vi "Update Map.vi"(8 "Direction":T1, 9 "Action":T2, 10 "Old Position":T4, 11 "Map in":T3[][](array[typedef])) -> (3 "Map out":T3[][](array[typedef]))   [LabVIEW 2020, in "Common.lvlib"]
uses:
  Common.lvlib
  Position.ctl
  Location Data.ctl
  Type Defs/Action Enum.ctl
  Type Defs/Direction Enum.ctl
  SubVIs/Read-Only Globals.vi
  Square/Board Size.vi
  SubVIs/Globals (private).vi
  Square/Square.lvclass
  Type Defs/SB Type Defs.lvlib
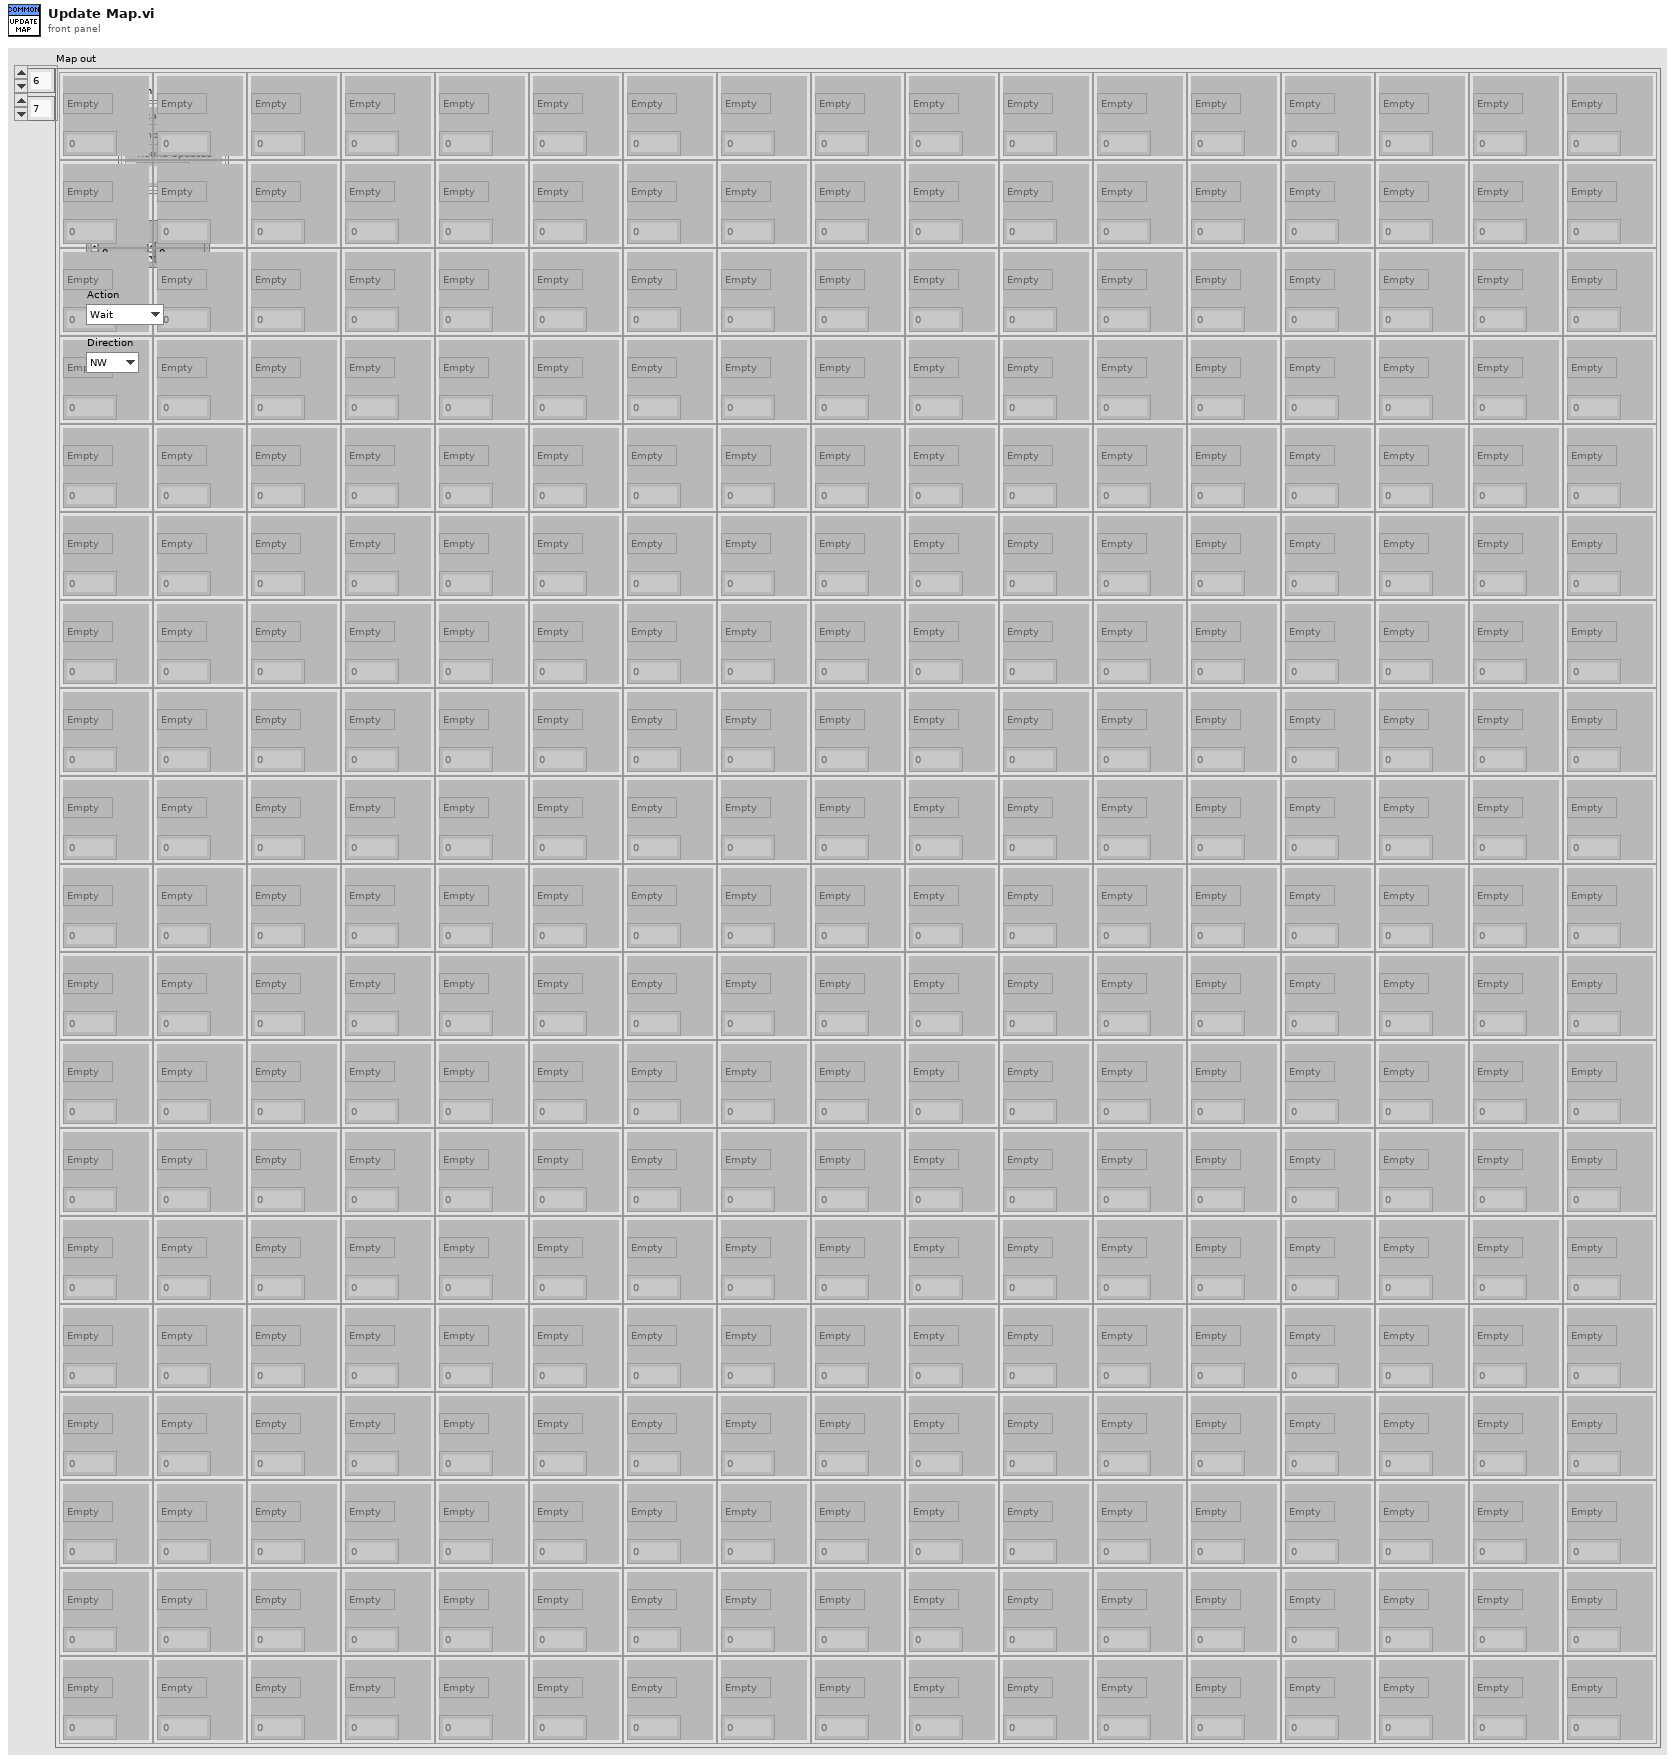
[diagram p1: front panel]
types:
  T1 = typedef "SB Type Defs.lvlib/Direction Enum.ctl" = enum16{"NW", "N", "NE", "E", "SE", "S", "SW", "W"}
  T2 = typedef "SB Type Defs.lvlib/Action Enum.ctl" = enum16{"Wait", "Move", "Attack", "Replicate"}
  T3 = typedef "Common.lvlib/Location Data.ctl" = cluster{"Location State":enum16{"Empty", "Enemy", "Attacked", "Occupied"}, "Round Updated":i32}
  T4 = typedef "Common.lvlib/Position.ctl" = cluster{"Column":i32, "Row":i32}
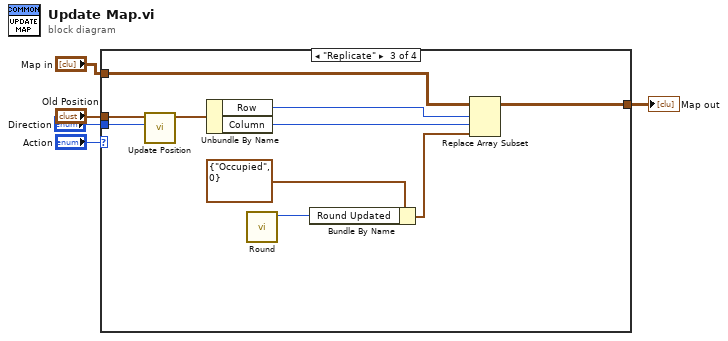
[diagram p0: block diagram]
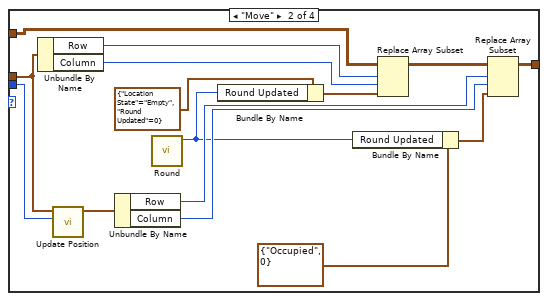
[diagram p3: hidden frame]
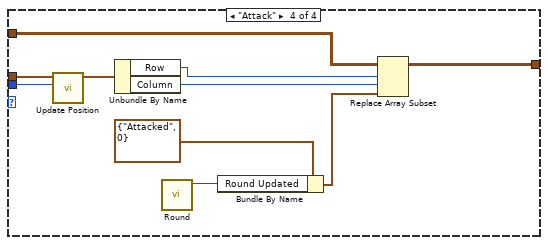
[diagram p4: hidden frame]
diagram:
  n1 = case shown="\"Replicate\"" "Action" {
    tunnel: "Old Position" -> [_ w11 w26 w36]
    tunnel: "Map in" -> [w6 w16 w29 w39]
    tunnel: [w6 w15 w28 w38] -> w3
    tunnel: "Direction" -> [_ w10 w24 w34]
    frame "Wait" {
    }
    frame "Move" {
      n2 = Unbundle By Name(w11) -> ("Row"=w21:i32, "Column"=w20:i32)
      n3 = call "Update Position.vi"("Direction"=w10, "Position in"=w11) -> ("Position out"=w12:T4)  [unwired: 9 in]
      n4 = Unbundle By Name(w12) -> ("Row"=w19:i32, "Column"=w18:i32)
      n5 = call "Round.vi"() -> ("Round"=w7:i32)  [unwired: 11 in]
      n6 = Bundle By Name(cluster=T3 {"Location State"=enum."Empty", "Round Updated"=0} ("new element/subarray"), "Round Updated"=w7) -> (w9:T3)
      n7 = Bundle By Name(cluster=T3 {"Location State"=enum."Occupied", "Round Updated"=0} ("new element/subarray"), "Round Updated"=w7) -> (w8:T3)
      n8 = Replace Array Subset(array=w16, new element=w9, index (row)=w21, index (col)=w20) -> (w17:T3[][])
      n9 = Replace Array Subset(array=w17, new element=w8, index (row)=w19, index (col)=w18) -> (w15:T3[][])
    }
    frame "Replicate" {
      n10 = call "Update Position.vi"("Direction"=w24, "Position in"=w26) -> ("Position out"=w25:T4)  [unwired: 9 in]
      n11 = Unbundle By Name(w25) -> ("Row"=w31:i32, "Column"=w30:i32)
      n12 = call "Round.vi"() -> ("Round"=w22:i32)  [unwired: 11 in]
      n13 = Bundle By Name(cluster=T3 {"Location State"=enum."Occupied", "Round Updated"=0} ("new element/subarray"), "Round Updated"=w22) -> (w23:T3)
      n14 = Replace Array Subset(array=w29, new element=w23, index (row)=w31, index (col)=w30) -> (w28:T3[][])
    }
    frame "Attack" {
      n15 = call "Update Position.vi"("Direction"=w34, "Position in"=w36) -> ("Position out"=w35:T4)  [unwired: 9 in]
      n16 = Unbundle By Name(w35) -> ("Row"=w41:i32, "Column"=w40:i32)
      n17 = call "Round.vi"() -> ("Round"=w32:i32)  [unwired: 11 in]
      n18 = Bundle By Name(cluster=T3 {"Location State"=enum."Attacked", "Round Updated"=0} ("new element/subarray"), "Round Updated"=w32) -> (w33:T3)
      n19 = Replace Array Subset(array=w39, new element=w33, index (row)=w41, index (col)=w40) -> (w38:T3[][])
    }
  }
  "Map out" <- w3
